vi "Set Number Of Connections To Make.vi"(8 "error in (no error)":errorcluster, 10 "Connections To Make":i32=-1, 11 "MultiplexedConnectionHandler in":refnum<class "MultiplexedConnectionHandler.lvclass">) -> (0 "error out":errorcluster, 3 "MultiplexedConnectionHandler out":refnum<class "MultiplexedConnectionHandler.lvclass">)   [LabVIEW 2019, in "MultiplexedConnectionHandler.lvlib" / "MultiplexedConnectionHandler.lvclass"]
uses:
  <vilib>/gpm_packages/@cs/Network-interface/Source/MultiplexedConnectionHandler/MultiplexedConnectionHandler/MultiplexedConnectionHandler.lvclass
  <vilib>/gpm_packages/@cs/Network-interface/Source/MultiplexedConnectionHandler/MultiplexedConnectionHandler/MultiplexedConnectionHandler.lvclass/MultiplexedConnectionHandler.ctl
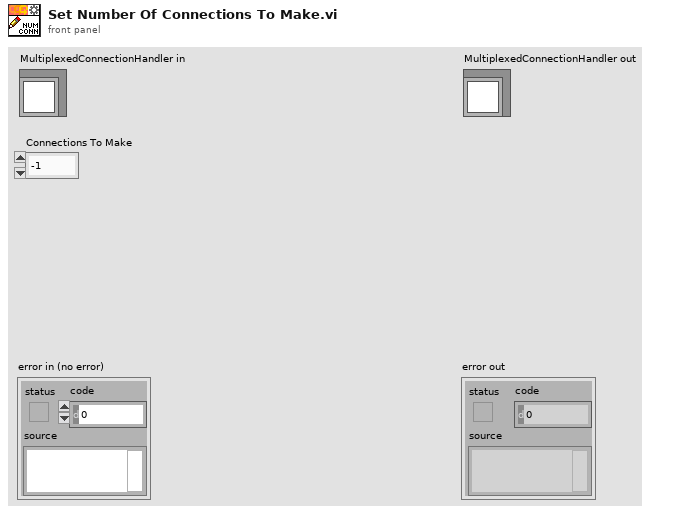
[diagram p1: front panel]
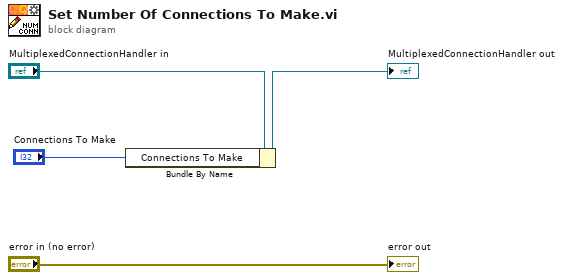
[diagram p0: block diagram]
diagram:
  n1 = Bundle By Name(cluster="MultiplexedConnectionHandler in", "Connections To Make"="Connections To Make") -> (→"MultiplexedConnectionHandler out":refnum<class "MultiplexedConnectionHandler.lvclass">)
  "error out" <- "error in (no error)"
